vi "PlotOHparams.vi"() -> ()   [LabVIEW 2014]
uses:
  TypeDefs/RectHatch.ctl
  TypeDefs/PowerSpeed.ctl
  <vilib>/Utility/file.llb/Read From Spreadsheet File (DBL).vi
panel:
  in  "DummyCube2":cluster{dbl, dbl}
  in  "DummyCubeLoc":cluster{dbl, dbl}
  in  "Save?":bool
  in  "Path":path
  in  "HighPower":dbl=1.0
  in  "Display":T1={"Mode"=enum."Inherit Value", "PointSize"=1.0, "LineWidth"=1.0}
  in  "LayerEnd":u32
  in  "LayerStart":u32
  in  "HatchPow":T2={"Power"=300.0, "Mark Speed"=400.0, "Jump Speed"=1000.0}
  in  "RectHatch":T3={"Width"=10.0, "Height"=10.0, "Angle"=45.0, "OffX"=0.1, "OffY"=0.1, "Spacing"=0.1} {"Spacing" format="%#_13g"; "OffY" format="%#_13g"; "OffX" format="%#_13g"; "Height" format="%#_13g"; "Width" format="%#_13g"}
  out "OH":T4(array[cluster])
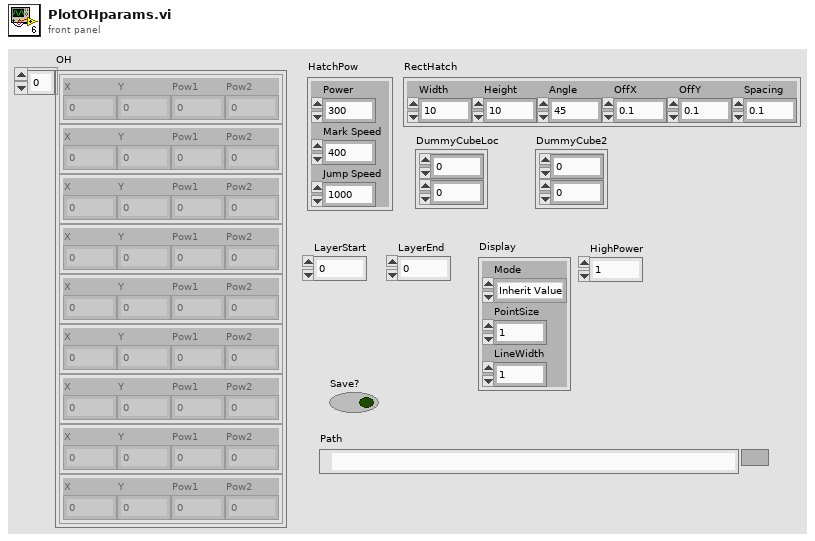
[diagram p1: front panel]
types:
  T1 = cluster{"Mode":enum16{"Inherit Value", "Points", "Wireframe", "Polygons"}, "PointSize":sgl, "LineWidth":sgl}
  T2 = typedef "PowerSpeed.ctl" = cluster{"Power":dbl, "Mark Speed":dbl, "Jump Speed":dbl}
  T3 = typedef "RectHatch.ctl" = cluster{"Width":dbl, "Height":dbl, "Angle":sgl, "OffX":dbl, "OffY":dbl, "Spacing":dbl}
  T4 = cluster{"X":dbl, "Y":dbl, "Pow1":dbl, "Pow2":dbl}[]
  T5 = typedef "PathSupreme.ctl" = cluster{"VelocityProfiles":T6[], "Path":T7}
  T6 = typedef "VelocityProfile.ctl" = cluster{"ID":u32, "Velocity":dbl, "Mode":string, "tV1":u32, "tV2":u32, "tL1":u32, "tL2":u32}
  T7 = typedef "PathCut.ctl" = cluster{"Type":string, "Tag":string, "Segments":T8[]}
  T8 = typedef "Segment.ctl" = cluster{"SegmentID":u16, "Power":sgl, "idxVelocityProfile":u16, "End":cluster{"X":sgl, "Y":sgl}}
  T9 = typedef "Point3D.ctl" = cluster{"X":sgl, "Y":sgl, "Z":sgl}
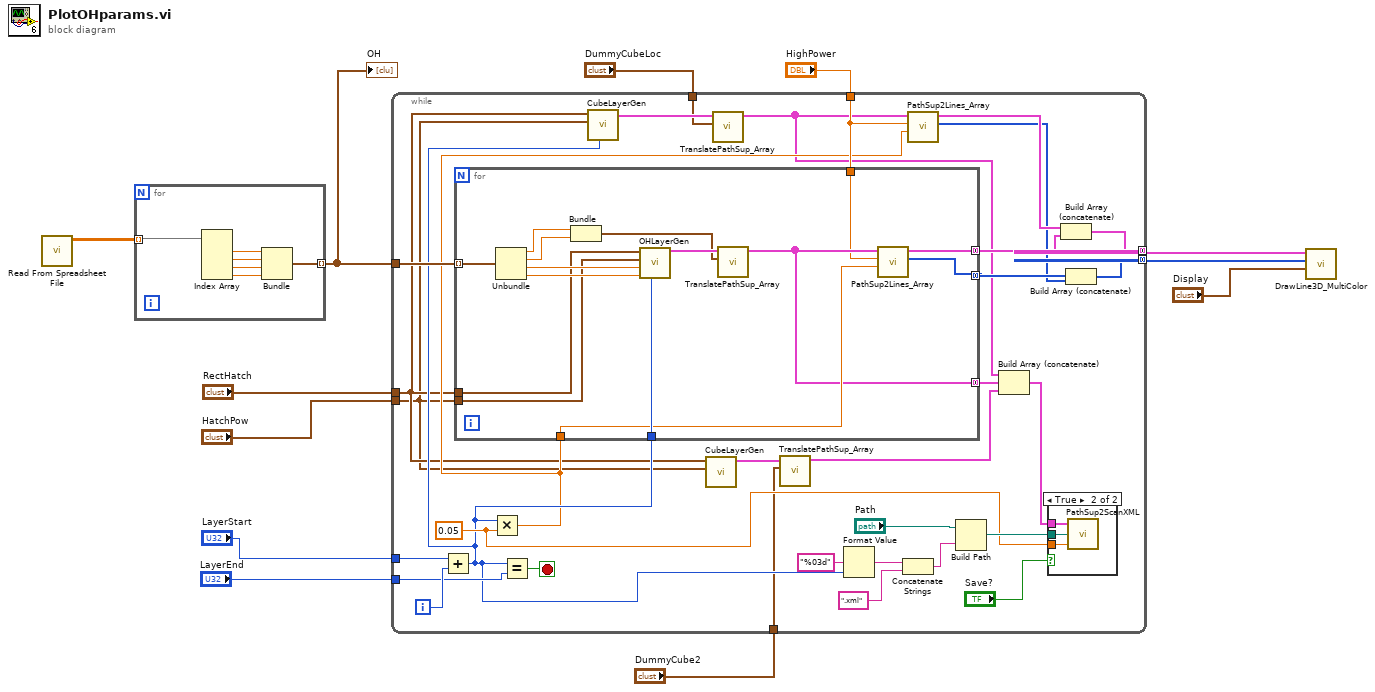
[diagram p0: block diagram]
diagram:
  n1 = call-poly <vilib>:"Read From Spreadsheet File.vi"() -> ("all rows"=w12:dbl[][])  [unwired: 7 in, 4 out]
  n2 = for {
    tunnel: w12 -> [w18] mode=indexing
    tunnel: [w13] -> w7 mode=indexing
    n3 = Index Array(array=w18) -> (element #1=w16:dbl, element #2=w17:dbl, element #3=w15:dbl, element #4=w14:dbl)  [unwired: 4 in]
    n4 = Bundle(w16, w17, w15, w14) -> (w13:cluster{dbl, dbl, dbl, dbl})  [unwired: 1 in]
  }
  "OH" <- w7
  n5 = while {
    tunnel: "HighPower" -> [w34]
    tunnel: [w30] -> w10 mode=concatenating
    tunnel: [w27] -> w9 mode=concatenating
    tunnel: w7 -> [w48]
    tunnel: "RectHatch" -> [w23]
    tunnel: "HatchPow" -> [w22]
    tunnel: "LayerEnd" -> [w47]
    tunnel: "LayerStart" -> [w46]
    tunnel: "DummyCubeLoc" -> [w35]
    tunnel: "DummyCube2" -> [w20]
    i -> [w50]
    stop <- w49 stop-if-true
    w39 = 0.05 ("y")
    n6 = Add(x=w46, y=w50) -> (x+y=w37:u32)
    n7 = Multiply(x=w37, y=w39) -> (x*y=w33:dbl)
    n8 = for {
      tunnel: w37 -> [w68]
      tunnel: w33 -> [w59]
      tunnel: w34 -> [w55]
      tunnel: [w67] -> w31 mode=concatenating
      tunnel: w48 -> [w66] mode=indexing
      tunnel: w23 -> [w63]
      tunnel: w22 -> [w62]
      tunnel: [w56] -> w26 mode=concatenating
      tunnel: [w54] -> w29 mode=concatenating
      n9 = Unbundle(w66) -> (w61:dbl, w60:dbl, w65:dbl, w64:dbl)
      n10 = Bundle(w61, w60) -> (w57:cluster{dbl, dbl})  [unwired: 1 in]
      n11 = call "OHLayerGen.vi"("Layer"=w68, "OHL2pow"=w64, "OHL1pow"=w65, "HatchPow"=w62, "RectHatch"=w63) -> ("PathSups"=w58:T5[])  [unwired: 6 in]
      n12 = call "TranslatePathSup_Array.vi"("Offset"=w57, "PathSupsIn"=w58) -> ("PathSupsOut"=w56:T5[])  [unwired: 9 in]
      n13 = call "PathSup2Lines_Array.vi"("Z"=w59, "HighPower"=w55, "PathSupIn"=w56) -> ("Colors"=w54:u32[], "Lines"=w67:cluster{"P0":T9, "P1":T9}[])  [unwired: 7 in]
    }
    n14 = Equal?(x=w37, y=w47) -> (x = y?=w49:bool)
    n15 = call "CubeLayerGen.vi"("Layer"=w37, "HatchPow"=w22, "RectHatch"=w23) -> ("PathSups"=w36:T5[])  [unwired: 8 in]
    n16 = call "CubeLayerGen.vi"("HatchPow"=w22, "RectHatch"=w23) -> ("PathSups"=w21:T5[])  [unwired: 9 in]
    n17 = call "TranslatePathSup_Array.vi"("Offset"=w35, "PathSupsIn"=w36) -> ("PathSupsOut"=w25:T5[])  [unwired: 9 in]
    n18 = call "TranslatePathSup_Array.vi"("Offset"=w20, "PathSupsIn"=w21) -> ("PathSupsOut"=w19:T5[])  [unwired: 9 in]
    n19 = Format Value(format string="%03d", value (0)=w37) -> (output string=w44:string)  [unwired: 1 in]
    n20 = Concatenate Strings(w44, ".xml" ("string")) -> (w42:string)
    n21 = call "PathSup2Lines_Array.vi"("Z"=w33, "HighPower"=w34, "PathSupIn"=w25) -> ("Colors"=w28:u32[], "Lines"=w32:cluster{"P0":T9, "P1":T9}[])  [unwired: 7 in]
    n22 = Build Path(base path="Path", name or relative path=w42) -> (appended path=w40:path)
    n23 = Build Array (concatenate)(w25, w26, w19) -> (w24:T5[])
    n24 = case shown="True" "Save?" {
      tunnel: w24 -> [_ w53]
      tunnel: w40 -> [_ w52]
      tunnel: w39 -> [_ w51]
      frame False {
      }
      frame True {
        n25 = call "PathSup2ScanXML.vi"("Thickness"=w51, "Path"=w52, "PathSupremes"=w53) -> ()  [unwired: 2 in, 1 out]
      }
    }
    n26 = Build Array (concatenate)(w32, w31) -> (w30:cluster{"P0":T9, "P1":T9}[])
    n27 = Build Array (concatenate)(w29, w28) -> (w27:u32[])
  }
  n28 = call "DrawLine3D_MultiColor.vi"("Display"="Display", "Colors"=w9, "Lines"=w10) -> ()  [unwired: 9 in]
